vi "PQgetssl.vi"(7 "error in (no error)":errorcluster, 10 "conn":u32) -> (0 "error out":errorcluster, 2 "ssl":u32, 3 "conn_out":u32)   [LabVIEW 2019, in "libpqlv.lvlib"]
doc: "Returns the SSL structure used in the connection, or null if SSL is not in use.\n\nSSL *PQgetssl(const PGconn *conn);\n\nThis structure can be used to verify encryption levels, check server certificates, and more. Refer to the OpenSSL documentation for information about this structure.\n\nYou must define USE_SSL in order to get the correct prototype for this function. Doing this will also automatically include ssl.h from OpenSSL."
uses:
  libpqlv.lvlib
  libpq.dll
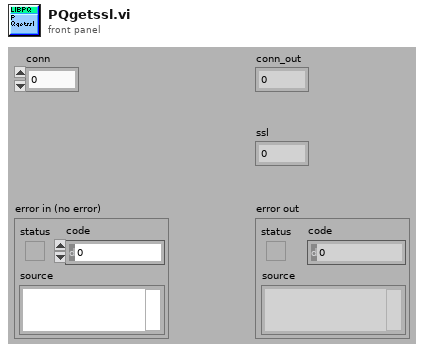
[diagram p1: front panel]
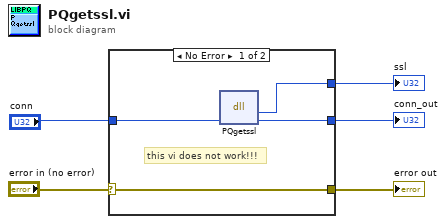
[diagram p0: block diagram]
diagram:
  n1 = case shown="No Error" "error in (no error)" {
    selector: "error in (no error)" -> [w9 w11]
    tunnel: [w9 w11] -> w4
    tunnel: [w8 _] -> w3
    tunnel: "conn" -> [w7 w10]
    tunnel: [w6 w10] -> w1
    frame No Error {
      # "this vi does not work!!!"
      n2 = dll-call lib="libpq.*" fn="PQgetssl"("conn"=w7) -> ("ssl"=w8:u32, "conn"=w6:u32)  [unwired: 3 in, 2 out]
    }
    frame Error {
    }
  }
  "ssl" <- w3
  "error out" <- w4
  "conn_out" <- w1
